vi "Check If Valid.vi"(11 "Actor API in":refnum<class "Actor API.lvclass">) -> (3 "Valid":bool)   [LabVIEW 2015, in "Actor API.lvclass"]
uses:
  Actor API.lvclass
  Actor API.lvclass/Actor API.ctl
  Messaging/Messenger/Messenger.lvclass
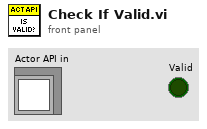
[diagram p1: front panel]
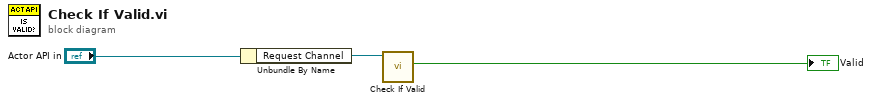
[diagram p0: block diagram]
diagram:
  n1 = Unbundle By Name("Actor API in") -> ("Request Channel"=w1:refnum<class "Messenger.lvclass">)
  n2 = call "Check If Valid.vi"("Messenger - Actor in"=w1) -> ("Is Valid"=→"Valid":bool)  [unwired: 8 in, 2 out]
